vi "Arduino Test.vi"() -> ()   [LabVIEW 2014]
uses:
  Type Defs/VL6180X DEFS.ctl
  <vilib>/Analysis/baseanly.llb/Mean (DBL).vi
  <vilib>/MakerHub/LINX/Public/Utilities/Open Serial.vi
  <vilib>/MakerHub/LINX/LMH-LINX.lvlib
  <vilib>/Analysis/NI_AALBase.lvlib
panel:
  in  "Serial Port - Arduino":refnum<visa-resource-name>="COM5"
  out "Loop Rate (Hz)":u32
  out "Data out":u8 format="%02x"
  out "range":dbl
  out "Array":dbl[](array[numeric])
  out "min value":dbl
  out "max value":dbl
  out "mean":dbl format="%0.2f"
  in  "Samples to Avg":i32=5
  in  "milliseconds to wait":u32=20
  out "Sensor Error Code":u8
  in  "Stop":bool
  out "Distance":cluster{"Distance (mm)":u8, u8}(graph)
  # "0 = No error\n6 = early convergence estimate check failed\n7 = max convergence issue"
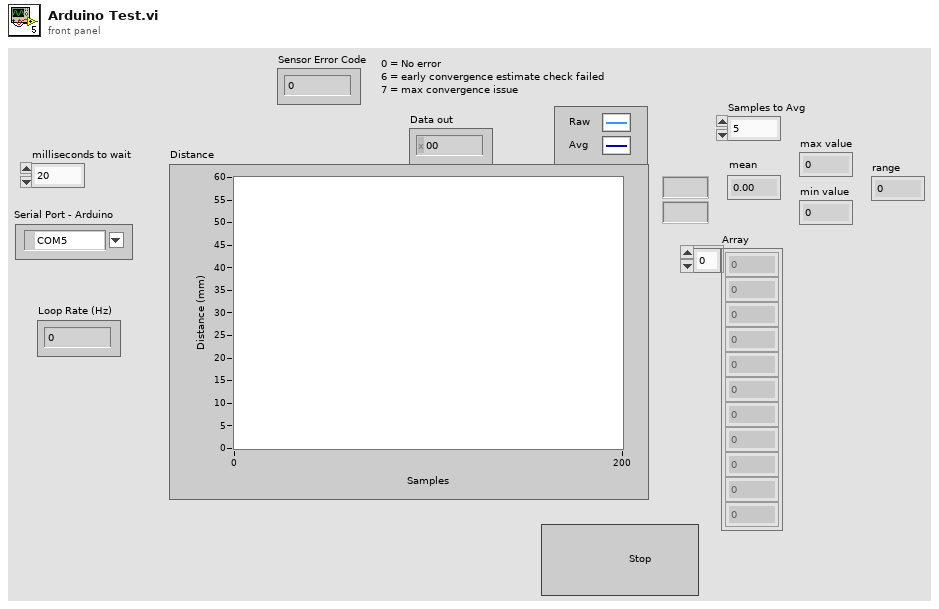
[diagram p1: front panel]
types:
  T1 = typedef "LMH-LINX.lvlib/LINX Ref.ctl" = cluster{"IO":T2, "Interface":T3, "LINX Device Config":T4}
  T2 = typedef "LMH-LINX.lvlib/Platform.ctl" = enum16{"Remote", "Local"}
  T3 = typedef "LMH-LINX.lvlib/Interface.ctl" = enum16{"Serial", "TCP"}
  T4 = typedef "LMH-LINX.lvlib/Device.lvlib/LINX Device Config.ctl" = cluster{"Interface":T3, "COM Port":refnum<visa-resource-name>, "TCP Configuration":T5, "Device Family":u8, "Device ID":u8, "Device Name":string, "TCP Ref":refnum<k5>, "Channels":T6}
  T5 = typedef "LMH-LINX.lvlib/Device.lvlib/TCP Config.ctl" = cluster{"IP Address":string, "Port":u16}
  T6 = typedef "LMH-LINX.lvlib/Channels.ctl" = cluster{"DI":u8[], "DO":u8[], "AI":u8[], "AO":u8[], "PWM":u8[], "QE":u8[], "UART":u8[], "I2C 2":u8[], "SPI":u8[], "CAN":u8[], "Servo":u8[], "AI Ref (V)":dbl, "AI Resolution (Bits)":u8, "AO Ref (V)":dbl, "AO Resolution (Bits)":u8}
  T7 = typedef "VL6180 Resource.ctl" = cluster{"LINX Resource":T1, "I2C Channel":u8, "I2C Slave Address":u8}
  T8 = typedef "VL6180X DEFS.ctl" = u16
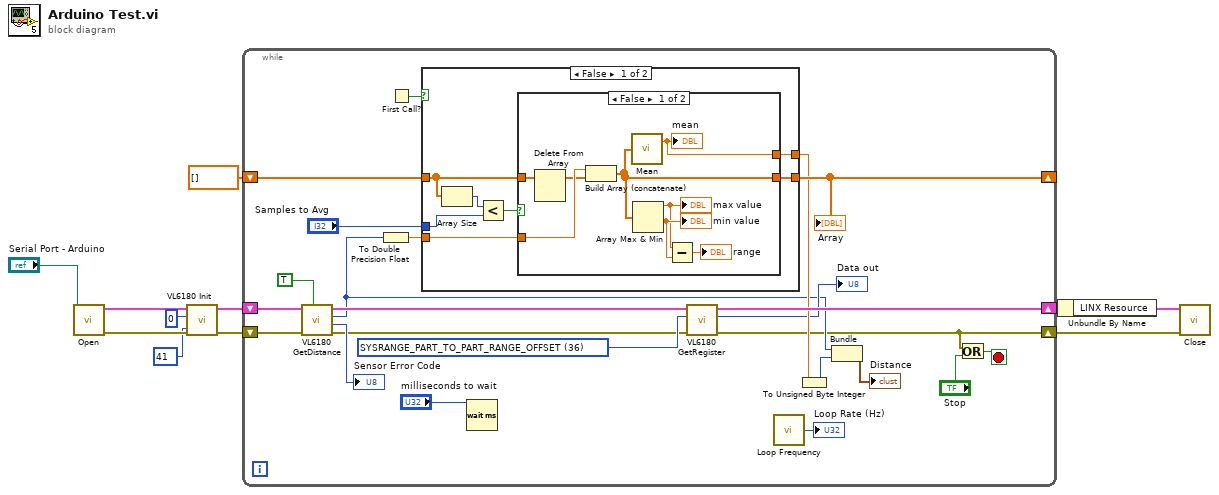
[diagram p0: block diagram]
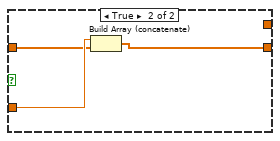
[diagram p2: hidden frame]
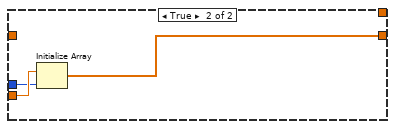
[diagram p3: hidden frame]
diagram:
  n1 = call-poly <vilib>:"Open.vi"("Serial Port"="Serial Port - Arduino") -> ("Error Out"=w10:errorcluster, "LINX Resource"=w11:T1)  [unwired: 8 in, 1 out]
  n2 = call "VL6180 Init.vi"("Error In"=w10, "I2C Slave Address (0)"=u8 41, "I2C Channel"=u8 0, "LINX Resource"=w11) -> ("Error Out"=w6:errorcluster, "VL6180 Resource"=w7:T7)  [unwired: 6 in]
  n3 = while {
    shift-right: [w25] -> w4
    shift-left: w7 -> [w34]
    shift-right: [w12] -> w5
    shift-left: w6 -> [w33]
    shift-right: [w27] -> _
    shift-left: dbl[] [] -> [w26]
    stop <- w13 stop-if-true
    w24 = T8 36 items=["IDENTIFICATION_MODEL_ID"=0, "IDENTIFICATION_MODEL_REV_MAJOR"=1, "IDENTIFICATION_MODEL_REV_MINOR"=2, "IDENTIFICATION_MODULE_REV_MAJOR"=3, "IDENTIFICATION_MODULE_REV_MINOR"=4, "IDENTIFICATION_DATE"=6, "IDENTIFICATION_TIME"=8, "SYSTEM_MODE_GPIO0"=16, "SYSTEM_MODE_GPIO1"=17, "SYSTEM_HISTORY_CTRL"=18, "SYSTEM_INTERRUPT_CONFIG_GPIO"=20, "SYSTEM_INTERRUPT_CLEAR"=21, "SYSTEM_FRESH_OUT_OF_RESET"=22, "SYSTEM_GROUPED_PARAMETER_HOLD"=23, "SYSRANGE_START"=24, "SYSRANGE_THRESH_HIGH"=25, "SYSRANGE_THRESH_LOW"=26, "SYSRANGE_INTERMEASUREMENT_PERIOD"=27, "SYSRANGE_MAX_CONVERGENCE_TIME"=28, "SYSRANGE_CROSSTALK_COMPENSATION_RATE"=30, "SYSRANGE_CROSSTALK_VALID_HEIGHT"=33, "SYSRANGE_EARLY_CONVERGENCE_ESTIMATE"=34, "SYSRANGE_PART_TO_PART_RANGE_OFFSET"=36, "SYSRANGE_RANGE_IGNORE_VALID_HEIGHT"=37, "SYSRANGE_RANGE_IGNORE_THRESHOLD"=38, "SYSRANGE_MAX_AMBIENT_LEVEL_MULT"=44, "SYSRANGE_RANGE_CHECK_ENABLES"=45, "SYSRANGE_VHV_RECALIBRATE"=46, "SYSRANGE_VHV_REPEAT_RATE"=49, "SYSALS_START"=56, "SYSALS_THRESH_HIGH"=58, "SYSALS_THRESH_LOW"=60, "SYSALS_INTERMEASUREMENT_PERIOD"=62, "SYSALS_ANALOGUE_GAIN"=63, "SYSALS_INTEGRATION_PERIOD"=64, "RESULT_RANGE_STATUS"=77, "RESULT_ALS_STATUS"=78, "RESULT_INTERRUPT_STATUS_GPIO"=79, "RESULT_ALS_VAL"=80, "RESULT_HISTORY_BUFFER"=82, "RESULT_RANGE_VAL"=98, "RESULT_RANGE_RAW"=100, "RESULT_RANGE_RETURN_RATE"=102, "RESULT_RANGE_REFERENCE_RATE"=104, "RESULT_RANGE_RETURN_SIGNAL_COUNT"=108, "RESULT_RANGE_REFERENCE_SIGNAL_COUNT"=112, "RESULT_RANGE_RETURN_AMB_COUNT"=116, "RESULT_RANGE_REFERENCE_AMB_COUNT"=120, "RESULT_RANGE_RETURN_CONV_TIME"=124, "RESULT_RANGE_REFERENCE_CONV_TIME"=128, "READOUT_AVERAGING_SAMPLE_PERIOD"=266, "FIRMWARE_BOOTUP"=281, "FIRMWARE_RESULT_SCALER"=288, "I2C_SLAVE_DEVICE_ADDRESS"=530, "INTERLEAVED_MODE_ENABLE"=675] ("VL6180X Constants")
    n4 = call "VL6180 GetDistance.vi"("Speed Read"=TRUE, "error in (no error)"=w33, "VL6180 Resource in"=w34) -> ("error out"=w22:errorcluster, "Sensor Error Code"=→"Sensor Error Code":u8, "Distance (mm)"=w16:u8, "VL6180 Resource out"=w23:T7)  [unwired: 5 in]
    n5 = To Double Precision Float(number=w16) -> (double precision float=w29:dbl)
    n6 = First Call?() -> (First Call?: T/F=w30:bool)
    n7 = case shown="False" w30 {
      tunnel: w29 -> [w38 w55]
      tunnel: "Samples to Avg" -> [w39 w54]
      tunnel: [w36 w53] -> w27
      tunnel: w26 -> [w37 _]
      tunnel: [w35 _] -> w19
      frame False {
        n8 = Array Size(array=w37) -> (size(s)=w40:i32)
        n9 = Less?(x=w40, y=w39) -> (x < y?=w41:bool)
        n10 = case shown="False" w41 {
          tunnel: w38 -> [w48 w52]
          tunnel: w37 -> [w49 w51]
          tunnel: [w46 w50] -> w36
          tunnel: [w42 _] -> w35
          frame False {
            n11 = Delete From Array(array=w49) -> (array with subset deleted=w47:dbl[])  [unwired: 2 in, 1 out]
            n12 = Build Array (concatenate)(w48, w47) -> (w46:dbl[])
            n13 = call-poly <vilib>:"Mean.vi"("X"=w46) -> ("mean"=w42:dbl)  [unwired: 1 out]
            "mean" <- w42
            n14 = Array Max & Min(array=w46) -> (max value=w44:dbl, min value=w45:dbl)  [unwired: 2 out]
            "max value" <- w44
            "min value" <- w45
            n15 = Subtract(x=w44, y=w45) -> (x-y=→"range":dbl)
          }
          frame True {
            n16 = Build Array (concatenate)(w52, w51) -> (w50:dbl[])
          }
        }
      }
      frame True {
        n17 = Initialize Array(w55, w54) -> (w53:dbl[])
      }
    }
    "Array" <- w27
    n18 = Wait (ms)(milliseconds to wait="milliseconds to wait") -> ()  [unwired: 1 out]
    n19 = call "VL6180 GetRegister.vi"("error in"=w22, "VL6180X Constants"=w24, "VL6180 Resource"=w23) -> ("error out"=w12:errorcluster, "Data out"=→"Data out":u8, "VL6180 Resource"=w25:T7)  [unwired: 6 in]
    n20 = call <vilib>:"Loop Frequency.vi"() -> ("Loop Rate (Hz)"=→"Loop Rate (Hz)":u32)
    n21 = To Unsigned Byte Integer(number=w19) -> (unsigned 8bit integer=w18:u8)
    n22 = Bundle("Distance (mm)"=w16, w18) -> (→"Distance":cluster{"Distance (mm)":u8, u8})  [unwired: 1 in]
    n23 = Or(x=w12, y="Stop") -> (x .or. y?=w13:bool)
  }
  n24 = Unbundle By Name(w4) -> ("LINX Resource"=w3:T1)
  n25 = call <vilib>:"Close.vi"("Error In"=w5, "LINX Resource"=w3) -> ()  [unwired: 9 in, 1 out]
